vi "Validate Configuration Metadata.vi"(8 "error in (no error)":errorcluster) -> (0 "error out":errorcluster, 2 "Invalid Parameters":string, 3 "Is Metadata Valid":bool)   [LabVIEW 2020, in "NI-DMM Measurement.lvlib"]
uses:
  NI-DMM Measurement.lvlib
  Measurement Configuration.ctl
  <vilib>/Utility/Data Type/NI_Data Type.lvlib
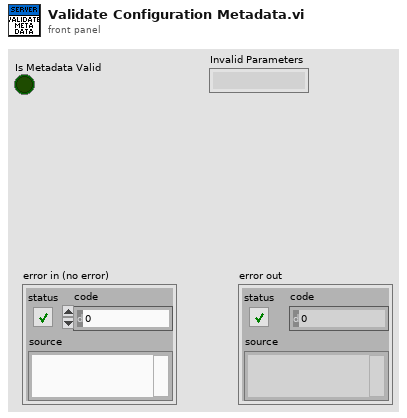
[diagram p1: front panel]
types:
  T1 = typedef "NI-DMM Measurement.lvlib/Measurement Configuration.ctl" = cluster{"Array in":dbl[]}
  T2 = typedef "NI-DMM Measurement.lvlib/Parameter Type Specialization.ctl" = cluster{"Parameter Name":string, "Type Specialization":T3, "Annotations":cluster{"Key":T4, "Value":string}[]}
  T3 = typedef "NI-DMM Measurement.lvlib/Type Specialization.ctl" = enum16{"none", "pin"}
  T4 = typedef "NI-DMM Measurement.lvlib/Key.ctl" = enum16{"none", "pin.instrument_type"}
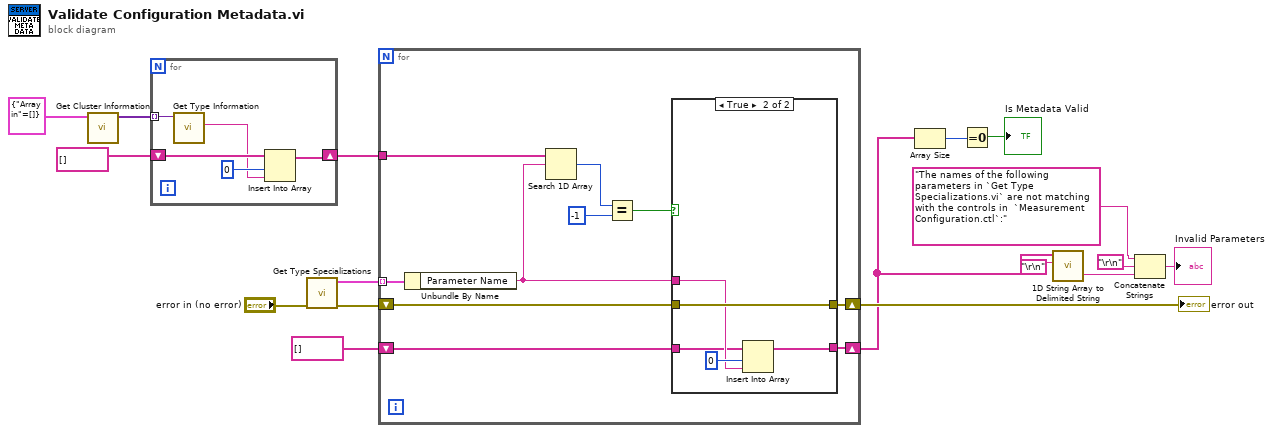
[diagram p0: block diagram]
diagram:
  n1 = call <vilib>:"Get Cluster Information.vi"("variant"=T1 {"Array in"=[]} ("Measurement Configuration")) -> ("cluster elements"=w13:variant[])  [unwired: 9 in, 1 out]
  n2 = for {
    tunnel: w13 -> [w22] mode=indexing
    shift-right: [w18] -> w11
    shift-left: string[] [] -> [w20]
    n3 = call <vilib>:"Get Type Information.vi"("variant"=w22) -> ("name"=w19:string)  [unwired: 6 in, 4 out]
    n4 = Insert Into Array(array=w20, index=0, new element=w19) -> (w18:string[])
  }
  n5 = call "Get Type Specializations.vi"("error in (no error)"="error in (no error)") -> ("error out"=w15:errorcluster, "Type Specializations"=w16:T2[])  [unwired: 9 in]
  n6 = for {
    tunnel: w16 -> [w32] mode=indexing
    shift-right: [w26] -> w9
    shift-left: w15 -> [w27]
    tunnel: w11 -> [w31]
    shift-right: [w23] -> w2
    shift-left: string[] [] -> [w25]
    n7 = Unbundle By Name(w32) -> ("Parameter Name"=w24:string)
    n8 = Search 1D Array(1D array=w31, element=w24) -> (index of element=w30:i32)  [unwired: 1 in]
    n9 = Equal?(x=w30, y=-1) -> (x = y?=w28:bool)
    n10 = case shown="True" w28 {
      tunnel: w27 -> [w34 w39]
      tunnel: [w34 w39] -> w26
      tunnel: w25 -> [w33 w36]
      tunnel: w24 -> [_ w37]
      tunnel: [w33 w35] -> w23
      frame False {
      }
      frame True {
        n11 = Insert Into Array(array=w36, index=0, new element=w37) -> (w35:string[])
      }
    }
  }
  "error out" <- w9
  n12 = Array Size(array=w2) -> (size(s)=w8:i32)
  n13 = Equal To 0?(x=w8) -> (x = 0?=→"Is Metadata Valid":bool)
  n14 = call <vilib>:"1D String Array to Delimited String.vi"("delimiter"="\r\n", "string array"=w2) -> ("delimited string"=w3:string)  [unwired: 9 in]
  n15 = Concatenate Strings("The names of the following parameters in `Get Type Specializations.vi` are not matching with the controls in  `Measurement Configuration.ctl`:" ("string"), "\r\n", w3) -> (→"Invalid Parameters":string)
